vi "RSNRPZ Get Initiate Continuous State.vi"(8 "error in (no error)":errorcluster, 10 "Channel (1)":i32=1, 11 "VISA session":refnum<visa-resource-name> caption="VISA resource name") -> (0 "error out":errorcluster, 2 "Continuous Initiate":bool, 3 "dup VISA session":refnum<visa-resource-name> caption="VISA resource name")   [LabVIEW 2010]
doc: "This VI returns whether single-shot or continuous (free-running) measurement is selected.\n\nRemote-control command(s):\nINIT:CONT?"
uses:
  rsnrpz_32.dll
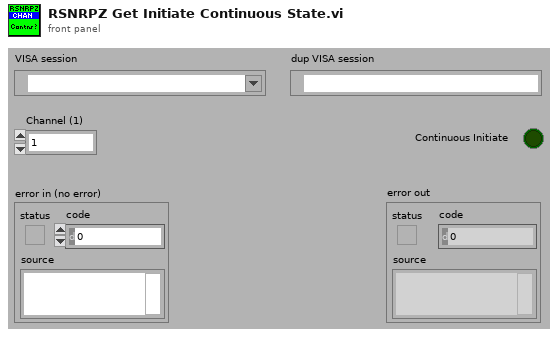
[diagram p1: front panel]
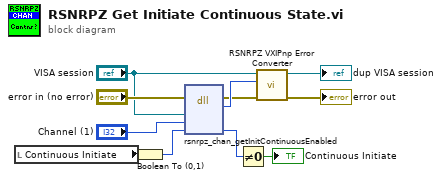
[diagram p0: block diagram]
diagram:
  n1 = local read "Continuous Initiate"() -> (w9:bool)
  n2 = Boolean To (0,1)(Boolean=w9) -> (0, 1=w7:i16)
  n3 = dll-call lib="rsnrpz_32.dll" fn="rsnrpz_chan_getInitContinuousEnabled"(error in="error in (no error)", "VISA Session"="VISA session", "Channel"="Channel (1)", "Continuous Initiate"=w7) -> (error out=w5:errorcluster, "Status"=w11:i32, "Continuous Initiate"=w8:u16)  [unwired: 4 in, 1 out]
  n4 = Not Equal To 0?(x=w8) -> (x != 0?=→"Continuous Initiate":bool)
  n5 = call <instrlib>:"RSNRPZ VXIPnp Error Converter.vi"("error in"=w5, "VXIPnp error code"=w11, "VISA session"="VISA session") -> ("error out"=→"error out":errorcluster, "dup VISA session"=→"dup VISA session":refnum<visa-resource-name>)  [unwired: 7 in]
